vi "rsidr_core_global.vi"() -> ()   [LabVIEW 2020, in "Rohde&Schwarz CMWXP NR FR1 Measurement.lvlib"] (continued)
"Help"="Queries the parameter 'AdditionalSpectrumEmission', signaled to the UE if the value is not OFF.\n\nSyntax:\n[CONFigure:]SIGNaling:NRADio:CELL:RFSettings:ASEMission? <CellName>\n\n<CellName>\nString\n\nAvailable Repeated Capabilities:\nNone\n\nRemote-control command(s):\n[CONFigure:]SIGNaling:NRADio:CELL:RFSettings:ASEMission?"}, {"Level"=4, "Class Only"=FALSE, "Identifier"="RSCMWXPNRFR1M_ATTR_SIGNALING_DUPLEX_MODE", "Descriptive Name"="Signaling Duplex Mode", "Data Type"=enum."RawString", "Command"="SIGN:NRAD:CELL:RFS:DMOD", "Access"=enum."Write Only", "Range Table"="", "Read Callback"="", "Write Callback"="", "Range Callback"="", "Check Callback"="", "Rngtable Callback"="", "Coerce Callback"="", "Supported Models"="", "Instrument Options"="", "Check Status Callback"="", "Flags"=0, "Help"="Selects the duplex mode.\n\nSyntax:\n[CONFigure:]SIGNaling:NRADio:CELL:RFSettings:DMODe <CellName>, <Duplexmode>\n\n<DuplexMode>\nValid Values:\nFDD\nTDD\n\nAvailable Repeated Capabilities:\nNone\n\nRemote-control command(s):\n[CONFigure:]SIGNaling:NRADio:CELL:RFSettings:DMODe"}, {"Level"=4, "Class Only"=FALSE, "Identifier"="RSCMWXPNRFR1M_ATTR_HIDDEN_QUERY_SIGNALING_DUPLEX_MODE", "Descriptive Name"="Query Signaling Duplex Mode", "Data Type"=enum."ViInt32", "Command"="SIGN:NRAD:CELL:RFS:DMOD?", "Access"=enum."Read Only", "Range Table"="rsCmwxpNrFr1M_rngDuplexMode", "Read Callback"="", "Write Callback"="", "Range Callback"="", "Check Callback"="", "Rngtable Callback"="", "Coerce Callback"="", "Supported Models"="", "Instrument Options"="", "Check Status Callback"="", "Flags"=8, "Help"="Queries the duplex mode.\n\nSyntax:\n[CONFigure:]SIGNaling:NRADio:CELL:RFSettings:DMODe? <CellName>\n\nParameters:\n<CellName>\n\nResponse:\n<DuplexMode>\nValid Values:\nFDD\nTDD\n\nAvailable Repeated Capabilities:\nNone\n\nRemote-control command(s):\n[CONFigure:]SIGNaling:NRADio:CELL:RFSettings:DMODe?"}, {"Level"=4, "Class Only"=TRUE, "Identifier"="", "Descriptive Name"="RF Settings", "Data Type"=enum."ViInt32", "Command"="", "Access"=enum."Read Only", "Range Table"="", "Read Callback"="", "Write Callback"="", "Range Callback"="", "Check Callback"="", "Rngtable Callback"="", "Coerce Callback"="", "Supported Models"="", "Instrument Options"="", "Check Status Callback"="", "Flags"=0, "Help"="Contains attributes for Signaling RF Settings."}, {"Level"=5, "Class Only"=FALSE, "Identifier"="RSCMWXPNRFR1M_ATTR_SIGNALING_RF_FREQUENCY_BAND_INDICATOR", "Descriptive Name"="Signaling RF Frequency Band Indicator", "Data Type"=enum."RawString", "Command"="SIGN:NRAD:CELL:RFS:FBIN", "Access"=enum."Write Only", "Range Table"="", "Read Callback"="", "Write Callback"="", "Range Callback"="", "Check Callback"="", "Rngtable Callback"="", "Coerce Callback"="", "Supported Models"="", "Instrument Options"="", "Check Status Callback"="", "Flags"=0, "Help"="Defines the frequency band.\n\nSyntax:\n[CONFigure:]SIGNaling:NRADio:CELL:RFSettings:FBINdicator <CellName>, <Fbi>\n\nAvailable Repeated Capabilities:\nNone\n\nRemote-control command(s):\n[CONFigure:]SIGNaling:NRADio:CELL:RFSettings:FBINdicator"}, {"Level"=5, "Class Only"=FALSE, "Identifier"="RSCMWXPNRFR1M_ATTR_HIDDEN_QUERY_SIGNALING_RF_FREQUENCY_BAND_INDICATOR", "Descriptive Name"="Query Signaling RF Frequency Band Indicator", "Data Type"=enum."ViInt32", "Command"="SIGN:NRAD:CELL:RFS:FBIN?", "Access"=enum."Read Only", "Range Table"="", "Read Callback"="", "Write Callback"="", "Range Callback"="", "Check Callback"="", "Rngtable Callback"="", "Coerce Callback"="", "Supported Models"="", "Instrument Options"="", "Check Status Callback"="", "Flags"=8, "Help"="Queries the frequency band.\n\nSyntax:\n[CONFigure:]SIGNaling:NRADio:CELL:RFSettings:FBINdicator? <CellName>\n\nParameters:\n<CellName>\nString\n\nAvailable Repeated Capabilities:\nNone\n\nRemote-control command(s):\n[CONFigure:]SIGNaling:NRADio:CELL:RFSettings:FBINdicator?"}, {"Level"=5, "Class Only"=FALSE, "Identifier"="RSCMWXPNRFR1M_ATTR_SIGNALING_RF_SUBCARRIER_SPACING", "Descriptive Name"="Signaling RF Subcarrier Spacing", "Data Type"=enum."RawString", "Command"="SIGN:NRAD:CELL:RFS:SSP", "Access"=enum."Write Only", "Range Table"="", "Read Callback"="", "Write Callback"="", "Range Callback"="", "Check Callback"="", "Rngtable Callback"="", "Coerce Callback"="", "Supported Models"="", "Instrument Options"="", "Check Status Callback"="", "Flags"=0, "Help"="Selects the subcarrier spacing.\n\nSyntax:\n[CONFigure:]SIGNaling:NRADio:CELL:RFSettings:SSPacing <CellName>, <Spacing>\n\nAvailable Repeated Capabilities:\nNone\n\nRemote-control command(s):\n[CONFigure:]SIGNaling:NRADio:CELL:RFSettings:SSPacing"}, {"Level"=5, "Class Only"=FALSE, "Identifier"="RSCMWXPNRFR1M_ATTR_HIDDEN_QUERY_SIGNALING_RF_SUBCARRIER_SPACING", "Descriptive Name"="Query Signaling RF Subcarrier Spacing", "Data Type"=enum."ViInt32", "Command"="SIGN:NRAD:CELL:RFS:SSP?", "Access"=enum."Read Only", "Range Table"="", "Read Callback"="", "Write Callback"="", "Range Callback"="", "Check Callback"="", "Rngtable Callback"="", "Coerce Callback"="", "Supported Models"="", "Instrument Options"="", "Check Status Callback"="", "Flags"=8, "Help"="Queries the subcarrier spacing.\n\nSyntax:\n[CONFigure:]SIGNaling:NRADio:CELL:RFSettings:SSPacing? <CellName>\n\nParameters:\n<CellName>\nString\n\nAvailable Repeated Capabilities:\nNone\n\nRemote-control command(s):\n[CONFigure:]SIGNaling:NRADio:CELL:RFSettings:SSPacing?"}, {"Level"=5, "Class Only"=FALSE, "Identifier"="RSCMWXPNRFR1M_ATTR_SIGNALING_RF_UL_CHANNEL_NUMBER_A", "Descriptive Name"="Signaling RF UL Channel Number A", "Data Type"=enum."RawString", "Command"="SIGN:NRAD:CELL:RFS:UL:APO:ARFC", "Access"=enum."Write Only", "Range Table"="", "Read Callback"="", "Write Callback"="", "Range Callback"="", "Check Callback"="", "Rngtable Callback"="", "Coerce Callback"="", "Supported Models"="", "Instrument Options"="", "Check Status Callback"="", "Flags"=0, "Help"="Sets the user-defined channel number of point A, for the uplink.\n\nSyntax:\n[CONFigure:]SIGNaling:NRADio:CELL:RFSettings:UL:APOint:ARFCn <CellName>, <Number>\n\nAvailable Repeated Capabilities:\nNone\n\nRemote-control command(s):\n[CONFigure:]SIGNaling:NRADio:CELL:RFSettings:UL:APOint:ARFCn"}, {"Level"=5, "Class Only"=FALSE, "Identifier"="RSCMWXPNRFR1M_ATTR_HIDDEN_QUERY_SIGNALING_RF_UL_CHANNEL_NUMBER_A", "Descriptive Name"="Query Signaling RF UL Channel Number A", "Data Type"=enum."ViInt32", "Command"="SIGN:NRAD:CELL:RFS:UL:APO:ARFC?", "Access"=enum."Read Only", "Range Table"="", "Read Callback"="", "Write Callback"="", "Range Callback"="", "Check Callback"="", "Rngtable Callback"="", "Coerce Callback"="", "Supported Models"="", "Instrument Options"="", "Check Status Callback"="", "Flags"=0, "Help"="Queries the user-defined channel number of point A, for the uplink.\n\nSyntax:\n[CONFigure:]SIGNaling:NRADio:CELL:RFSettings:UL:APOint:ARFCn? <CellName>\n\nParameters:\n<CellName>\nString\n\nAvailable Repeated Capabilities:\nNone\n\nRemote-control command(s):\n[CONFigure:]SIGNaling:NRADio:CELL:RFSettings:UL:APOint:ARFCn?"}, {"Level"=5, "Class Only"=FALSE, "Identifier"="RSCMWXPNRFR1M_ATTR_SIGNALING_RF_UL_FREQUENCY_A", "Descriptive Name"="Signaling RF UL Frequency A", "Data Type"=enum."RawString", "Command"="SIGN:NRAD:CELL:RFS:UL:APO:FREQ", "Access"=enum."Write Only", "Range Table"="", "Read Callback"="", "Write Callback"="", "Range Callback"="", "Check Callback"="", "Rngtable Callback"="", "Coerce Callback"="", "Supported Models"="", "Instrument Options"="", "Check Status Callback"="", "Flags"=0, "Help"="Sets the user-defined frequency of point A, for the uplink.\n\nSyntax:\n[CONFigure:]SIGNaling:NRADio:CELL:RFSettings:UL:APOint:FREQuency <CellName>, <Frequency>\n\nAvailable Repeated Capabilities:\nNone\n\nRemote-control command(s):\n[CONFigure:]SIGNaling:NRADio:CELL:RFSettings:UL:APOint:FREQuency"}, {"Level"=5, "Class Only"=FALSE, "Identifier"="RSCMWXPNRFR1M_ATTR_HIDDEN_QUERY_SIGNALING_RF_UL_FREQUENCY_A", "Descriptive Name"="Query Signaling RF UL Frequency A", "Data Type"=enum."ViReal64", "Command"="SIGN:NRAD:CELL:RFS:UL:APO:FREQ?", "Access"=enum."Read Only", "Range Table"="", "Read Callback"="", "Write Callback"="", "Range Callback"="", "Check Callback"="", "Rngtable Callback"="", "Coerce Callback"="", "Supported Models"="", "Instrument Options"="", "Check Status Callback"="", "Flags"=8, "Help"="Queries the user-defined frequency of point A, for the uplink.\n\nSyntax:\n[CONFigure:]SIGNaling:NRADio:CELL:RFSettings:UL:APOint:FREQuency? <CellName>\n\nParameters:\n<CellName>\nString\n\nAvailable Repeated Capabilities:\nNone\n\nRemote-control command(s):\n[CONFigure:]SIGNaling:NRADio:CELL:RFSettings:UL:APOint:FREQuency?"}, {"Level"=5, "Class Only"=FALSE, "Identifier"="RSCMWXPNRFR1M_ATTR_SIGNALING_RF_UL_LOCATION_A", "Descriptive Name"="Signaling RF UL Location A", "Data Type"=enum."RawString", "Command"="SIGN:NRAD:CELL:RFS:UL:APO:LOC", "Access"=enum."Write Only", "Range Table"="", "Read Callback"="", "Write Callback"="", "Range Callback"="", "Check Callback"="", "Rngtable Callback"="", "Coerce Callback"="", "Supported Models"="", "Instrument Options"="", "Check Status Callback"="", "Flags"=0, "Help"="Selects a method for defining the frequency of point A, for the uplink.\n\nSyntax:\n[CONFigure:]SIGNaling:NRADio:CELL:RFSettings:UL:APOint:LOCation <CellName>, <Location>\n\n<Location>\nAutomatic selection of mid, low or high position in the frequency band.\nValid Values:\nMID\nLOW\nHIGH\nUSER - User-defined frequency, specified via separate command.\n\nAvailable Repeated Capabilities:\nNone\n\nRemote-control command(s):\n[CONFigure:]SIGNaling:NRADio:CELL:RFSettings:UL:APOint:LOCation"}, {"Level"=5, "Class Only"=FALSE, "Identifier"="RSCMWXPNRFR1M_ATTR_HIDDEN_QUERY_SIGNALING_RF_UL_LOCATION_A", "Descriptive Name"="Query Signaling RF UL Location A", "Data Type"=enum."ViInt32", "Command"="SIGN:NRAD:CELL:RFS:UL:APO:LOC?", "Access"=enum."Read Only", "Range Table"="rsCmwxpNrFr1M_rngLocation", "Read Callback"="", "Write Callback"="", "Range Callback"="", "Check Callback"="", "Rngtable Callback"="", "Coerce Callback"="", "Supported Models"="", "Instrument Options"="", "Check Status Callback"="", "Flags"=8, "Help"="Queries a method for defining the frequency of point A, for the uplink.\n\nSyntax:\n[CONFigure:]SIGNaling:NRADio:CELL:RFSettings:UL:APOint:LOCation? <CellName>\n\nParameters:\n<CellName>\nString\n\nResponse:\n<Location>\nAutomatic selection of mid, low or high position in the frequency band.\nValid Values:\nMID\nLOW\nHIGH\nUSER - User-defined frequency, specified via separate command.\n\nAvailable Repeated Capabilities:\nNone\n\nRemote-control command(s):\n[CONFigure:]SIGNaling:NRADio:CELL:RFSettings:UL:APOint:LOCation?"}, {"Level"=5, "Class Only"=FALSE, "Identifier"="RSCMWXPNRFR1M_ATTR_SIGNALING_RF_UL_BANDWIDTH", "Descriptive Name"="Signaling RF UL Bandwidth", "Data Type"=enum."RawString", "Command"="SIGN:NRAD:CELL:RFS:UL:BWID", "Access"=enum."Write Only", "Range Table"="", "Read Callback"="", "Write Callback"="", "Range Callback"="", "Check Callback"="", "Rngtable Callback"="", "Coerce Callback"="", "Supported Models"="", "Instrument Options"="", "Check Status Callback"="", "Flags"=0, "Help"="Selects the channel bandwidth for the uplink.\n\nSyntax:\n[CONFigure:]SIGNaling:NRADio:CELL:RFSettings:UL:BWIDth <CellName>, <Bandwidth>\n\n<Bandwidth>\nNumeric value in Hz or enumerated value in MHz.\nValid Values:\nnumeric | B005 | B010 | B015 | B020 | B025 | B030 | B040 | B050 | B060 | B070 | B080 | B090 | B100\n\nAvailable Repeated Capabilities:\nNone\n\nRemote-control command(s):\n[CONFigure:]SIGNaling:NRADio:CELL:RFSettings:UL:BWIDth"}, {"Level"=5, "Class Only"=FALSE, "Identifier"="RSCMWXPNRFR1M_ATTR_HIDDEN_QUERY_SIGNALING_RF_UL_BANDWIDTH", "Descriptive Name"="Query Signaling RF UL Bandwidth", "Data Type"=enum."ViInt32", "Command"="SIGN:NRAD:CELL:RFS:UL:BWID?", "Access"=enum."Read Only", "Range Table"="rsCmwxpNrFr1M_rngChannelBandwidth", "Read Callback"="", "Write Callback"="", "Range Callback"="", "Check Callback"="", "Rngtable Callback"="", "Coerce Callback"="", "Supported Models"="", "Instrument Options"="", "Check Status Callback"="", "Flags"=8, "Help"="Queries the channel bandwidth for the uplink.\n\nSyntax:\n[CONFigure:]SIGNaling:NRADio:CELL:RFSettings:UL:BWIDth? <CellName>\n\nParameters:\n<CellName>\n\nResponse:\n<Bandwidth>\nNumeric value in Hz or enumerated value in MHz.\nValid Values:\nnumeric | B005 | B010 | B015 | B020 | B025 | B030 | B040 | B050 | B060 | B070 | B080 | B090 | B100\n\nAvailable Repeated Capabilities:\nNone\n\nRemote-control command(s):\n[CONFigure:]SIGNaling:NRADio:CELL:RFSettings:UL:BWIDth?"}, {"Level"=4, "Class Only"=TRUE, "Identifier"="", "Descriptive Name"="TDD", "Data Type"=enum."ViInt32", "Command"="", "Access"=enum."Read Only", "Range Table"="", "Read Callback"="", "Write Callback"="", "Range Callback"="", "Check Callback"="", "Rngtable Callback"="", "Coerce Callback"="", "Supported Models"="", "Instrument Options"="", "Check Status Callback"="", "Flags"=0, "Help"="Contains attributes for TDD Signaling."}, {"Level"=5, "Class Only"=FALSE, "Identifier"="RSCMWXPNRFR1M_ATTR_SIGNALING_TDD_DL_FLEXIBLE_SLOT_SYMBOL", "Descriptive Name"="Signaling TDD DL Flexible Slot Symbol", "Data Type"=enum."RawString", "Command"="SIGN:NRAD:CELL:TDD:PATT{Pattern}:DL:FSSY", "Access"=enum."Write Only", "Range Table"="", "Read Callback"="", "Write Callback"="", "Range Callback"="", "Check Callback"="", "Rngtable Callback"="", "Coerce Callback"="", "Supported Models"="", "Instrument Options"="", "Check Status Callback"="", "Flags"=0, "Help"="Defines the number of DL symbols in the flexible slot of the UL-DL pattern <p>.\n\nSyntax:\n[CONFigure:]SIGNaling:NRADio:CELL:TDD:PATTern<p>:DL:FSSYmbol <CellName>, <Symbol>\n\nAvailable Repeated Capabilities:\nPattern: p1\r\n\nRemote-control command(s):\n[CONFigure:]SIGNaling:NRADio:CELL:TDD:PATTern<p>:DL:FSSYmbol"}, {"Level"=5, "Class Only"=FALSE, "Identifier"="RSCMWXPNRFR1M_ATTR_HIDDEN_QUERY_SIGNALING_TDD_DL_FLEXIBLE_SLOT_SYMBOL", "Descriptive Name"="Query Signaling TDD DL Flexible Slot Symbol", "Data Type"=enum."ViInt32", "Command"="SIGN:NRAD:CELL:TDD:PATT{Pattern}:DL:FSSY?", "Access"=enum."Read Only", "Range Table"="", "Read Callback"="", "Write Callback"="", "Range Callback"="", "Check Callback"="", "Rngtable Callback"="", "Coerce Callback"="", "Supported Models"="", "Instrument Options"="", "Check Status Callback"="", "Flags"=8, "Help"="Queries the number of DL symbols in the flexible slot of the UL-DL pattern <p>.\n\nSyntax:\n[CONFigure:]SIGNaling:NRADio:CELL:TDD:PATTern<p>:DL:FSSYmbol? <CellName>\n\nParameters:\n<CellName>\nString\n\nAvailable Repeated Capabilities:\nPattern: p1\r\n\nRemote-control command(s):\n[CONFigure:]SIGNaling:NRADio:CELL:TDD:PATTern<p>:DL:FSSYmbol?"}, {"Level"=5, "Class Only"=FALSE, "Identifier"="RSCMWXPNRFR1M_ATTR_SIGNALING_TDD_DL_SLOTS", "Descriptive Name"="Signaling TDD DL Slots", "Data Type"=enum."RawString", "Command"="SIGN:NRAD:CELL:TDD:PATT{Pattern}:DL:NSL", "Access"=enum."Write Only", "Range Table"="", "Read Callback"="", "Write Callback"="", "Range Callback"="", "Check Callback"="", "Rngtable Callback"="", "Coerce Callback"="", "Supported Models"="", "Instrument Options"="", "Check Status Callback"="", "Flags"=0, "Help"="Defines the number of DL slots in the UL-DL pattern <p>.\n\nSyntax:\n[CONFigure:]SIGNaling:NRADio:CELL:TDD:PATTern<p>:DL:NSLots <CellName>, <Number>\n\nAvailable Repeated Capabilities:\nPattern: p1\r\n\nRemote-control command(s):\n[CONFigure:]SIGNaling:NRADio:CELL:TDD:PATTern<p>:DL:NSLots"}, {"Level"=5, "Class Only"=FALSE, "Identifier"="RSCMWXPNRFR1M_ATTR_HIDDEN_QUERY_SIGNALING_TDD_DL_SLOTS", "Descriptive Name"="Query Signaling TDD DL Slots", "Data Type"=enum."ViInt32", "Command"="SIGN:NRAD:CELL:TDD:PATT{Pattern}:DL:NSL?", "Access"=enum."Read Only", "Range Table"="", "Read Callback"="", "Write Callback"="", "Range Callback"="", "Check Callback"="", "Rngtable Callback"="", "Coerce Callback"="", "Supported Models"="", "Instrument Options"="", "Check Status Callback"="", "Flags"=8, "Help"="Queries the number of DL slots in the UL-DL pattern <p>.\n\nSyntax:\n[CONFigure:]SIGNaling:NRADio:CELL:TDD:PATTern<p>:DL:NSLots? <CellName>\n\nParameters:\n<CellName>\nString\n\nAvailable Repeated Capabilities:\nPattern: p1\r\n\nRemote-control command(s):\n[CONFigure:]SIGNaling:NRADio:CELL:TDD:PATTern<p>:DL:NSLots?"}, {"Level"=5, "Class Only"=FALSE, "Identifier"="RSCMWXPNRFR1M_ATTR_SIGNALING_TDD_PERIODICITY", "Descriptive Name"="Signaling TDD Periodicity", "Data Type"=enum."RawString", "Command"="SIGN:NRAD:CELL:TDD:PATT{Pattern}:PER", "Access"=enum."Write Only", "Range Table"="", "Read Callback"="", "Write Callback"="", "Range Callback"="", "Check Callback"="", "Rngtable Callback"="", "Coerce Callback"="", "Supported Models"="", "Instrument Options"="", "Check Status Callback"="", "Flags"=0, "Help"="Configures the periodicity of the UL-DL pattern <p>.\n\nSyntax:\n[CONFigure:]SIGNaling:NRADio:CELL:TDD:PATTern<p>:PERiodicity <CellName>, <Periodicity>\n\n<Periodicity>\nPeriodicity, 0.5 ms (P0P5) to 10 ms (P10).\nValid Values:\nP0P5 | P0P6 | P1 | P1P2 | P2 | P2P5 | P3 | P4 | P5 | P10\n\nAvailable Repeated Capabilities:\nPattern: p1\r\n\nRemote-control command(s):\n[CONFigure:]SIGNaling:NRADio:CELL:TDD:PATTern<p>:PERiodicity"}, {"Level"=5, "Class Only"=FALSE, "Identifier"="RSCMWXPNRFR1M_ATTR_HIDDEN_QUERY_SIGNALING_TDD_PERIODICITY", "Descriptive Name"="Query Signaling TDD Periodicity", "Data Type"=enum."ViInt32", "Command"="SIGN:NRAD:CELL:TDD:PATT{Pattern}:PER?", "Access"=enum."Read Only", "Range Table"="rsCmwxpNrFr1M_rngTDDPeriodicity", "Read Callback"="", "Write Callback"="", "Range Callback"="", "Check Callback"="", "Rngtable Callback"="", "Coerce Callback"="", "Supported Models"="", "Instrument Options"="", "Check Status Callback"="", "Flags"=8, "Help"="Queries the periodicity of the UL-DL pattern <p>.\n\nSyntax:\n[CONFigure:]SIGNaling:NRADio:CELL:TDD:PATTern<p>:PERiodicity? <CellName>\n\nParameters:\n<CellName>\nString\n\nResponse:\n<Periodicity>\nPeriodicity, 0.5 ms (P0P5) to 10 ms (P10).\nValid Values:\nP0P5 | P0P6 | P1 | P1P2 | P2 | P2P5 | P3 | P4 | P5 | P10\n\nAvailable Repeated Capabilities:\nPattern: p1\r\n\nRemote-control command(s):\n[CONFigure:]SIGNaling:NRADio:CELL:TDD:PATTern<p>:PERiodicity?"}, {"Level"=5, "Class Only"=FALSE, "Identifier"="RSCMWXPNRFR1M_ATTR_SIGNALING_TDD_UL_FLEXIBLE_SLOT_SYMBOL", "Descriptive Name"="Signaling TDD UL Flexible Slot Symbol", "Data Type"=enum."RawString", "Command"="SIGN:NRAD:CELL:TDD:PATT{Pattern}:UL:FSSY", "Access"=enum."Write Only", "Range Table"="", "Read Callback"="", "Write Callback"="", "Range Callback"="", "Check Callback"="", "Rngtable Callback"="", "Coerce Callback"="", "Supported Models"="", "Instrument Options"="", "Check Status Callback"="", "Flags"=0, "Help"="Defines the number of UL symbols in the flexible slot of the UL-DL pattern <p>.\n\nSyntax:\n[CONFigure:]SIGNaling:NRADio:CELL:TDD:PATTern<p>:UL:FSSYmbol <CellName>, <Symbol>\n\nAvailable Repeated Capabilities:\nPattern: p1\r\n\nRemote-control command(s):\n[CONFigure:]SIGNaling:NRADio:CELL:TDD:PATTern<p>:UL:FSSYmbol"}, {"Level"=5, "Class Only"=FALSE, "Identifier"="RSCMWXPNRFR1M_ATTR_HIDDEN_QUERY_SIGNALING_TDD_UL_FLEXIBLE_SLOT_SYMBOL", "Descriptive Name"="Query Signaling TDD UL Flexible Slot Symbol", "Data Type"=enum."ViInt32", "Command"="SIGN:NRAD:CELL:TDD:PATT{Pattern}:UL:FSSY?", "Access"=enum."Read Only", "Range Table"="", "Read Callback"="", "Write Callback"="", "Range Callback"="", "Check Callback"="", "Rngtable Callback"="", "Coerce Callback"="", "Supported Models"="", "Instrument Options"="", "Check Status Callback"="", "Flags"=8, "Help"="Queries the number of UL symbols in the flexible slot of the UL-DL pattern <p>.\n\nSyntax:\n[CONFigure:]SIGNaling:NRADio:CELL:TDD:PATTern<p>:UL:FSSYmbol? <CellName>\n\nParameters:\n<CellName>\nString\n\nAvailable Repeated Capabilities:\nPattern: p1\r\n\nRemote-control command(s):\n[CONFigure:]SIGNaling:NRADio:CELL:TDD:PATTern<p>:UL:FSSYmbol?"}, {"Level"=5, "Class Only"=FALSE, "Identifier"="RSCMWXPNRFR1M_ATTR_SIGNALING_TDD_UL_SLOTS", "Descriptive Name"="Signaling TDD UL Slots", "Data Type"=enum."RawString", "Command"="SIGN:NRAD:CELL:TDD:PATT{Pattern}:UL:NSL", "Access"=enum."Write Only", "Range Table"="", "Read Callback"="", "Write Callback"="", "Range Callback"="", "Check Callback"="", "Rngtable Callback"="", "Coerce Callback"="", "Supported Models"="", "Instrument Options"="", "Check Status Callback"="", "Flags"=0, "Help"="Defines the number of UL slots in the UL-DL pattern <p>.\n\nSyntax:\n[CONFigure:]SIGNaling:NRADio:CELL:TDD:PATTern<p>:UL:NSLots <CellName>, <Number>\n\nAvailable Repeated Capabilities:\nPattern: p1\r\n\nRemote-control command(s):\n[CONFigure:]SIGNaling:NRADio:CELL:TDD:PATTern<p>:UL:NSLots"}, {"Level"=5, "Class Only"=FALSE, "Identifier"="RSCMWXPNRFR1M_ATTR_HIDDEN_QUERY_SIGNALING_TDD_UL_SLOTS", "Descriptive Name"="Query Signaling TDD UL Slots", "Data Type"=enum."ViInt32", "Command"="SIGN:NRAD:CELL:TDD:PATT{Pattern}:UL:NSL?", "Access"=enum."Read Only", "Range Table"="", "Read Callback"="", "Write Callback"="", "Range Callback"="", "Check Callback"="", "Rngtable Callback"="", "Coerce Callback"="", "Supported Models"="", "Instrument Options"="", "Check Status Callback"="", "Flags"=8, "Help"="Queries the number of UL slots in the UL-DL pattern <p>.\n\nSyntax:\n[CONFigure:]SIGNaling:NRADio:CELL:TDD:PATTern<p>:UL:NSLots? <CellName>\n\nParameters:\n<CellName>\nString\n\nAvailable Repeated Capabilities:\nPattern: p1\r\n\nRemote-control command(s):\n[CONFigure:]SIGNaling:NRADio:CELL:TDD:PATTern<p>:UL:NSLots?"}, {"Level"=3, "Class Only"=TRUE, "Identifier"="", "Descriptive Name"="PRACH Settings", "Data Type"=enum."ViInt32", "Command"="", "Access"=enum."Read Only", "Range Table"="", "Read Callback"="", "Write Callback"="", "Range Callback"="", "Check Callback"="", "Rngtable Callback"="", "Coerce Callback"="", "Supported Models"="", "Instrument Options"="", "Check Status Callback"="", "Flags"=0, "Help"="This class contains attributes that configure the PRACH settings."}, {"Level"=4, "Class Only"=FALSE, "Identifier"="RSCMWXPNRFR1M_ATTR_PRACH_CONFIGURATION_INDEX", "Descriptive Name"="PRACH Configuration Index", "Data Type"=enum."ViInt32", "Command"="CONF:NRS:MEAS{instance}:PRAC:PCIN", "Access"=enum."Read/Write", "Range Table"="rsCmwxpNrFr1M_rngPRACHConfigurationIndex", "Read Callback"="", "Write Callback"="", "Range Callback"="", "Check Callback"="", "Rngtable Callback"="", "Coerce Callback"="", "Supported Models"="", "Instrument Options"="", "Check Status Callback"="", "Flags"=0, "Help"="The PRACH configuration index identifies the PRACH configuration used by the UE (preamble format, which resources in the time domain are allowed for transmission of preambles etc.).\n\nAvailable Repeated Capabilities:\ninstance: i0, i1, i2, i3, i4, i5, i6, i7, i8, i9, i10, i11, i12, i13, i14, i15, i16, i17, i18, i19, i20, i21, i22, i23, i24, i25, i26, i27, i28, i29, i30, i31, i32\r\n\nRemote-control command(s):\nCONFigure:NRSub:MEAS<i>:PRACh:PCINdex"}, {"Level"=4, "Class Only"=FALSE, "Identifier"="RSCMWXPNRFR1M_ATTR_PRACH_SUBCARRIER_SPACING", "Descriptive Name"="PRACH Subcarrier Spacing", "Data Type"=enum."ViInt32", "Command"="CONF:NRS:MEAS{instance}:PRAC:SCSP", "Access"=enum."Read/Write", "Range Table"="rsCmwxpNrFr1M_rngPRACHSubcarrierSpacing", "Read Callback"="", "Write Callback"="", "Range Callback"="", "Check Callback"="", "Rngtable Callback"="", "Coerce Callback"="", "Supported Models"="", "Instrument Options"="", "Check Status Callback"="", "Flags"=0, "Help"="Specifies the subcarrier spacing used by the UE for the preambles. The allowed subset of values depends on the preamble format.\n\nAvailable Repeated Capabilities:\ninstance: i0, i1, i2, i3, i4, i5, i6, i7, i8, i9, i10, i11, i12, i13, i14, i15, i16, i17, i18, i19, i20, i21, i22, i23, i24, i25, i26, i27, i28, i29, i30, i31, i32\r\n\nRemote-control command(s):\nCONFigure:NRSub:MEAS<i>:PRACh:SCSPacing"}, {"Level"=4, "Class Only"=FALSE, "Identifier"="RSCMWXPNRFR1M_ATTR_PRACH_LOGICAL_ROOT_SEQUENCE", "Descriptive Name"="PRACH Logical Root Sequence", "Data Type"=enum."ViInt32", "Command"="CONF:NRS:MEAS{instance}:PRAC:LRS", "Access"=enum."Read/Write", "Range Table"="rsCmwxpNrFr1M_rngPRACHLogicalRootSequence", "Read Callback"="", "Write Callback"="", "Range Callback"="", "Check Callback"="", "Rngtable Callback"="", "Coerce Callback"="", "Supported Models"="", "Instrument Options"="", "Check Status Callback"="", "Flags"=0, "Help"="Specifies the logical root sequence index to be used for generation of the preamble sequence.\n\nAvailable Repeated Capabilities:\ninstance: i0, i1, i2, i3, i4, i5, i6, i7, i8, i9, i10, i11, i12, i13, i14, i15, i16, i17, i18, i19, i20, i21, i22, i23, i24, i25, i26, i27, i28, i29, i30, i31, i32\r\n\nRemote-control command(s):\nCONFigure:NRSub:MEAS<i>:PRACh:LRSindex"}, {"Level"=4, "Class Only"=FALSE, "Identifier"="RSCMWXPNRFR1M_ATTR_PRACH_ZERO_CORRELATION_ZONE", "Descriptive Name"="PRACH Zero Correlation Zone", "Data Type"=enum."ViInt32", "Command"="CONF:NRS:MEAS{instance}:PRAC:ZCZ", "Access"=enum."Read/Write", "Range Table"="rsCmwxpNrFr1M_rngPRACHZeroCorrelationZone", "Read Callback"="", "Write Callback"="", "Range Callback"="", "Check Callback"="", "Rngtable Callback"="", "Coerce Callback"="", "Supported Models"="", "Instrument Options"="", "Check Status Callback"="", "Flags"=0, "Help"="Specifies the zero correlation zone config, i.e. which NCS value of an NCS set is used for generation of the preamble sequence.\n\nAvailable Repeated Capabilities:\ninstance: i0, i1, i2, i3, i4, i5, i6, i7, i8, i9, i10, i11, i12, i13, i14, i15, i16, i17, i18, i19, i20, i21, i22, i23, i24, i25, i26, i27, i28, i29, i30, i31, i32\r\n\nRemote-control command(s):\nCONFigure:NRSub:MEAS<i>:PRACh:ZCZone"}, {"Level"=4, "Class Only"=FALSE, "Identifier"="RSCMWXPNRFR1M_ATTR_PRACH_FREQUENCY_OFFSET_ENABLED", "Descriptive Name"="PRACH Frequency Offset Enabled", "Data Type"=enum."ViBoolean", "Command"="CONF:NRS:MEAS{instance}:PRAC:PFOF:AUTO", "Access"=enum."Read/Write", "Range Table"="", "Read Callback"="", "Write Callback"="", "Range Callback"="", "Check Callback"="", "Rngtable Callback"="", "Coerce Callback"="", "Supported Models"="", "Instrument Options"="", "Check Status Callback"="", "Flags"=0, "Help"="Enables or disables automatic detection of the PRACH frequency offset.\n\nAvailable Repeated Capabilities:\ninstance: i0, i1, i2, i3, i4, i5, i6, i7, i8, i9, i10, i11, i12, i13, i14, i15, i16, i17, i18, i19, i20, i21, i22, i23, i24, i25, i26, i27, i28, i29, i30, i31, i32\r\n\nRemote-control command(s):\nCONFigure:NRSub:MEAS<i>:PRACh:PFOFfset:AUTO"}, {"Level"=4, "Class Only"=FALSE, "Identifier"="RSCMWXPNRFR1M_ATTR_PRACH_FREQUENCY_OFFSET", "Descriptive Name"="PRACH Frequency Offset", "Data Type"=enum."ViInt32", "Command"="CONF:NRS:MEAS{instance}:PRAC:PFOF", "Access"=enum."Read/Write", "Range Table"="", "Read Callback"="", "Write Callback"="", "Range Callback"="", "Check Callback"="", "Rngtable Callback"="", "Coerce Callback"="", "Supported Models"="", "Instrument Options"="", "Check Status Callback"="", "Flags"=0, "Help"="Specifies the PRACH frequency offset. This setting is only relevant if automatic detection is disabled.\n\nAvailable Repeated Capabilities:\ninstance: i0, i1, i2, i3, i4, i5, i6, i7, i8, i9, i10, i11, i12, i13, i14, i15, i16, i17, i18, i19, i20, i21, i22, i23, i24, i25, i26, i27, i28, i29, i30, i31, i32\r\n\nRemote-control command(s):\nCONFigure:NRSub:MEAS<i>:PRACh:PFOFfset"}, {"Level"=4, "Class Only"=FALSE, "Identifier"="RSCMWXPNRFR1M_ATTR_PRACH_SEQUENCE_INDEX_ENABLED", "Descriptive Name"="PRACH Sequence Index Enabled", "Data Type"=enum."ViBoolean", "Command"="CONF:NRS:MEAS{instance}:PRAC:SIND:AUTO", "Access"=enum."Read/Write", "Range Table"="", "Read Callback"="", "Write Callback"="", "Range Callback"="", "Check Callback"="", "Rngtable Callback"="", "Coerce Callback"="", "Supported Models"="", "Instrument Options"="", "Check Status Callback"="", "Flags"=0, "Help"="Enables or disables automatic detection of the sequence index.\n\nAvailable Repeated Capabilities:\ninstance: i0, i1, i2, i3, i4, i5, i6, i7, i8, i9, i10, i11, i12, i13, i14, i15, i16, i17, i18, i19, i20, i21, i22, i23, i24, i25, i26, i27, i28, i29, i30, i31, i32\r\n\nRemote-control command(s):\nCONFigure:NRSub:MEAS<i>:PRACh:SINDex:AUTO"}, {"Level"=4, "Class Only"=FALSE, "Identifier"="RSCMWXPNRFR1M_ATTR_PRACH_SEQUENCE_INDEX", "Descriptive Name"="PRACH Sequence Index", "Data Type"=enum."ViInt32", "Command"="CONF:NRS:MEAS{instance}:PRAC:SIND", "Access"=enum."Read/Write", "Range Table"="rsCmwxpNrFr1M_rngPRACHSequenceIndex", "Read Callback"="", "Write Callback"="", "Range Callback"="", "Check Callback"="", "Rngtable Callback"="", "Coerce Callback"="", "Supported Models"="", "Instrument Options"="", "Check Status Callback"="", "Flags"=0, "Help"="Specifies the sequence index, i.e. which of the 64 preamble sequences of the cell is used by the UE. This setting is only relevant if automatic detection is disabled.\n\nAvailable Repeated Capabilities:\ninstance: i0, i1, i2, i3, i4, i5, i6, i7, i8, i9, i10, i11, i12, i13, i14, i15, i16, i17, i18, i19, i20, i21, i22, i23, i24, i25, i26, i27, i28, i29, i30, i31, i32\r\n\nRemote-control command(s):\nCONFigure:NRSub:MEAS<i>:PRACh:SINDex"}, {"Level"=1, "Class Only"=TRUE, "Identifier"="", "Descriptive Name"="Multi Eval Meas", "Data Type"=enum."ViInt32", "Command"="", "Access"=enum."Read Only", "Range Table"="", "Read Callback"="", "Write Callback"="", "Range Callback"="", "Check Callback"="", "Rngtable Callback"="", "Coerce Callback"="", "Supported Models"="", "Instrument Options"="", "Check Status Callback"="", "Flags"=0, "Help"="The attributes for the NR FR1 multi-evaluation measurement are divided into the groups listed below. The general measurement settings also affect the measurement."}, {"Level"=2, "Class Only"=FALSE, "Identifier"="RSCMWXPNRFR1M_ATTR_NETWORK_SIGNALED_VALUE", "Descriptive Name"="Network Signaled Value", "Data Type"=enum."ViInt32", "Command"="CONF:NRS:MEAS{instance}:MEV:NSV", "Access"=enum."Read/Write", "Range Table"="rsCmwxpNrFr1M_rngNetworkSignaledValue", "Read Callback"="", "Write Callback"="", "Range Callback"="", "Check Callback"="", "Rngtable Callback"="", "Coerce Callback"="", "Supported Models"="", "Instrument Options"="", "Check Status Callback"="", "Flags"=0, "Help"="Selects the 'network signaled value'.\n\nAvailable Repeated Capabilities:\ninstance: i0, i1, i2, i3, i4, i5, i6, i7, i8, i9, i10, i11, i12, i13, i14, i15, i16, i17, i18, i19, i20, i21, i22, i23, i24, i25, i26, i27, i28, i29, i30, i31, i32\r\n\nRemote-control command(s):\nCONFigure:NRSub:MEAS<i>:MEValuation:NSValue"}, {"Level"=2, "Class Only"=FALSE, "Identifier"="RSCMWXPNRFR1M_ATTR_NRB_VIEW_FILTER_ENABLED", "Descriptive Name"="NRB View Filter Enabled", "Data Type"=enum."ViBoolean", "Command"="CONF:NRS:MEAS{instance}:MEV:NVF", "Access"=enum."Read/Write", "Range Table"="", "Read Callback"="", "Write Callback"="", "Range Callback"="", "Check Callback"="", "Rngtable Callback"="", "Coerce Callback"="", "Supported Models"="", "Instrument Options"="", "Check Status Callback"="", "Flags"=0, "Help"="Specifies, enables or disables the number of resource blocks (NRB) view filter. If the filter is active, only slots with a matching number of allocated resource blocks are measured.\n\nAvailable Repeated Capabilities:\ninstance: i0, i1, i2, i3, i4, i5, i6, i7, i8, i9, i10, i11, i12, i13, i14, i15, i16, i17, i18, i19, i20, i21, i22, i23, i24, i25, i26, i27, i28, i29, i30, i31, i32\r\n\nRemote-control command(s):\nCONFigure:NRSub:MEAS<i>:MEValuation:NVFilter"}, {"Level"=2, "Class Only"=FALSE, "Identifier"="RSCMWXPNRFR1M_ATTR_NRB_VIEW_FILTER", "Descriptive Name"="NRB View Filter", "Data Type"=enum."ViInt32", "Command"="CONF:NRS:MEAS{instance}:MEV:NVF", "Access"=enum."Read/Write", "Range Table"="", "Read Callback"="", "Write Callback"="", "Range Callback"="", "Check Callback"="", "Rngtable Callback"="", "Coerce Callback"="", "Supported Models"="", "Instrument Options"="", "Check Status Callback"="", "Flags"=0, "Help"="Specifies, enables or disables the number of resource blocks (NRB) view filter. If the filter is active, only slots with a matching number of allocated resource blocks are measured.\n\nAvailable Repeated Capabilities:\ninstance: i0, i1, i2, i3, i4, i5, i6, i7, i8, i9, i10, i11, i12, i13, i14, i15, i16, i17, i18, i19, i20, i21, i22, i23, i24, i25, i26, i27, i28, i29, i30, i31, i32\r\n\nRemote-control command(s):\nCONFigure:NRSub:MEAS<i>:MEValuation:NVFilter"}, {"Level"=2, "Class Only"=TRUE, "Identifier"="", "Descriptive Name"="Control and States", "Data Type"=enum."ViInt32", "Command"="", "Access"=enum."Read Only", "Range Table"="", "Read Callback"="", "Write Callback"="", "Range Callback"="", "Check Callback"="", "Rngtable Callback"="", "Coerce Callback"="", "Supported Models"="", "Instrument Options"="", "Check Status Callback"="", "Flags"=0, "Help"="Measurement control and states."}, {"Level"=3, "Class Only"=FALSE, "Identifier"="RSCMWXPNRFR1M_ATTR_MULTI_EVAL_MEAS_INIT", "Descriptive Name"="Multi Eval Meas Init", "Data Type"=enum."None", "Command"="INIT:NRS:MEAS{instance}:MEV", "Access"=enum."Write Only", "Range Table"="", "Read Callback"="", "Write Callback"="", "Range Callback"="", "Check Callback"="", "Rngtable Callback"="", "Coerce Callback"="", "Supported Models"="", "Instrument Options"="", "Check Status Callback"="", "Flags"=1, "Help"="Starts or restarts the measurement; the measurement enters the 'RUN' state.\n\nAvailable Repeated Capabilities:\ninstance: i0, i1, i2, i3, i4, i5, i6, i7, i8, i9, i10, i11, i12, i13, i14, i15, i16, i17, i18, i19, i20, i21, i22, i23, i24, i25, i26, i27, i28, i29, i30, i31, i32\r\n\nRemote-control command(s):\nINITiate:NRSub:MEAS<i>:MEValuation"}, {"Level"=3, "Class Only"=FALSE, "Identifier"="RSCMWXPNRFR1M_ATTR_MULTI_EVAL_MEAS_ABORT", "Descriptive Name"="Multi Eval Meas Abort", "Data Type"=enum."None", "Command"="ABOR:NRS:MEAS{instance}:MEV", "Access"=enum."Write Only", "Range Table"="", "Read Callback"="", "Write Callback"="", "Range Callback"="", "Check Callback"="", "Rngtable Callback"="", "Coerce Callback"="", "Supported Models"="", "Instrument Options"="", "Check Status Callback"="", "Flags"=0, "Help"="Causes a running measurement to stop immediately; the measurement enters the 'OFF' state. All measurement values are set to NAV. Allocated resources are released.\n\nAvailable Repeated Capabilities:\ninstance: i0, i1, i2, i3, i4, i5, i6, i7, i8, i9, i10, i11, i12, i13, i14, i15, i16, i17, i18, i19, i20, i21, i22, i23, i24, i25, i26, i27, i28, i29, i30, i31, i32\r\n\nRemote-control command(s):\nABORt:NRSub:MEAS<i>:MEValuation"}, {"Level"=3, "Class Only"=FALSE, "Identifier"="RSCMWXPNRFR1M_ATTR_MULTI_EVAL_MEAS_STOP", "Descriptive Name"="Multi Eval Meas Stop", "Data Type"=enum."None", "Command"="STOP:NRS:MEAS{instance}:MEV", "Access"=enum."Write Only", "Range Table"="", "Read Callback"="", "Write Callback"="", "Range Callback"="", "Check Callback"="", "Rngtable Callback"="", "Coerce Callback"="", "Supported Models"="", "Instrument Options"="", "Check Status Callback"="", "Flags"=0, "Help"="Causes a running measurement to stop immediately; the measurement enters the 'RDY' state. Measurement results are kept. The resources remain allocated to the measurement.\n\nAvailable Repeated Capabilities:\ninstance: i0, i1, i2, i3, i4, i5, i6, i7, i8, i9, i10, i11, i12, i13, i14, i15, i16, i17, i18, i19, i20, i21, i22, i23, i24, i25, i26, i27, i28, i29, i30, i31, i32\r\n\nRemote-control command(s):\nSTOP:NRSub:MEAS<i>:MEValuation"}, {"Level"=3, "Class Only"=FALSE, "Identifier"="RSCMWXPNRFR1M_ATTR_MULTI_EVAL_MEAS_MEASUREMENT_STATE", "Descriptive Name"="Multi Eval Meas Measurement State", "Data Type"=enum."RawString", "Command"="FETC:NRS:MEAS{instance}:MEV:STAT:ALL?", "Access"=enum."Read Only", "Range Table"="", "Read Callback"="", "Write Callback"="", "Range Callback"="", "Check Callback"="", "Rngtable Callback"="", "Coerce Callback"="", "Supported Models"="", "Instrument Options"="", "Check Status Callback"="", "Flags"=0, "Help"="Queries the main measurement state and the measurement substates. Both measurement substates are relevant for running measurements only. Use FETCh:...:STATe? to query the main measurement state only. Use INITiate..., STOP..., ABORt... to change the measurement state.\n\nAvailable Repeated Capabilities:\ninstance: i0, i1, i2, i3, i4, i5, i6, i7, i8, i9, i10, i11, i12, i13, i14, i15, i16, i17, i18, i19, i20, i21, i22, i23, i24, i25, i26, i27, i28, i29, i30, i31, i32\r\n\nRemote-control command(s):\nFETCh:NRSub:MEAS<i>:MEValuation:STATe:ALL?"}, {"Level"=2, "Class Only"=TRUE, "Identifier"="", "Descriptive Name"="Configuration", "Data Type"=enum."ViInt32", "Command"="", "Access"=enum."Read Only", "Range Table"="", "Read Callback"="", "Write Callback"="", "Range Callback"="", "Check Callback"="", "Rngtable Callback"="", "Coerce Callback"="", "Supported Models"="", "Instrument Options"="", "Check Status Callback"="", "Flags"=0, "Help"="Multi Evaluation measurement configuration attributes."}, {"Level"=3, "Class Only"=FALSE, "Identifier"="RSCMWXPNRFR1M_ATTR_ALL_RESULTS_ENABLED", "Descriptive Name"="All Results Enabled", "Data Type"=enum."RawString", "Command"="CONF:NRS:MEAS{instance}:MEV:RES", "Access"=enum."Read/Write", "Range Table"="", "Read Callback"="", "Write Callback"="", "Range Callback"="", "Check Callback"="", "Rngtable Callback"="", "Coerce Callback"="", "Supported Models"="", "Instrument Options"="", "Check Status Callback"="", "Flags"=0, "Help"="Enables or disables the evaluation of results in the multi-evaluation measurement. This command combines most other CONFigure:NRSub:MEAS<i>:MEValuation:RESult... commands.\n\nSyntax:\nCONFigure:NRSub:MEAS<i>:MEValuation:RESult[:ALL] <EVM>, <MagnitudeError>, <PhaseError>, <InbandEmissions>, <EVMversusC>, <IQ>, <EquSpecFlatness>, <TXMeasurement>, <SpecEmMask>, <ACLR>[, <PowerMonitor>, <PowerDynamics>]\n\n<EVM>\nValid Values:\nOFF\nON\n\n<MagnitudeError>\nValid Values:\nOFF\nON\n\n<PhaseError>\nValid Values:\nOFF\nON\n\n<InbandEmissions>\nValid Values:\nOFF\nON\n\n<EVMversusC>\nEVM vs. subcarrier\nValid Values:\nOFF\nON\n\n<IQ>\nIQ constellation diagram\nValid Values:\nOFF\nON\n\n<EquSpecFlatness>\nEqualizer spectrum flatness\nValid Values:\nOFF\nON\n\n<TXMeasurement>\nTX measurement statistical overview\nValid Values:\nOFF\nON\n\n<SpecEmMask>\nSpectrum emission mask\nValid Values:\nOFF\nON\n\n<ACLR>\nAdjacent channel leakage power ratio\nValid Values:\nOFF\nON\n\n<PowerMonitor>\nValid Values:\nOFF\nON\n\n<PowerDynamics>\nValid Values:\nOFF\nON\n\nAvailable Repeated Capabilities:\ninstance: i0, i1, i2, i3, i4, i5, i6, i7, i8, i9, i10, i11, i12, i13, i14, i15, i16, i17, i18, i19, i20, i21, i22, i23, i24, i25, i26, i27, i28, i29, i30, i31, i32\r\n\nRemote-control command(s):\nCONFigure:NRSub:MEAS<i>:MEValuation:RESult[:ALL]"}, {"Level"=3, "Class Only"=FALSE, "Identifier"="RSCMWXPNRFR1M_ATTR_MEASURE_SLOT", "Descriptive Name"="Measure Slot", "Data Type"=enum."ViInt32", "Command"="CONF:NRS:MEAS{instance}:MEV:MSL", "Access"=enum."Read/Write", "Range Table"="rsCmwxpNrFr1M_rngMeasureSlot", "Read Callback"="", "Write Callback"="", "Range Callback"="", "Check Callback"="", "Rngtable Callback"="", "Coerce Callback"="", "Supported Models"="", "Instrument Options"="", "Check Status Callback"="", "Flags"=0, "Help"="Selects which slots of the 'Measure Subframe' are measured.\n\nAvailable Repeated Capabilities:\ninstance: i0, i1, i2, i3, i4, i5, i6, i7, i8, i9, i10, i11, i12, i13, i14, i15, i16, i17, i18, i19, i20, i21, i22, i23, i24, i25, i26, i27, i28, i29, i30, i31, i32\r\n\nRemote-control command(s):\nCONFigure:NRSub:MEAS<i>:MEValuation:MSLot"}, {"Level"=3, "Class Only"=FALSE, "Identifier"="RSCMWXPNRFR1M_ATTR_SUBFRAMES_AND_SLOTS", "Descriptive Name"="Subframes And Slots", "Data Type"=enum."RawString", 
